vi "Test Collection.vi"(8 "error in (no error)":errorcluster) -> (0 "error out":errorcluster)   [LabVIEW 2020]
uses:
  cc2f4b2e-6b9b-4032-8eb1-861370e43379.vi
  70896fcf-518f-4248-9f1c-0e40431e55ec.vi
  c8c48edb-c7f5-472d-977d-3a0b36aefcc9.vi
  3ab85443-7e8d-4878-a956-06c51692e772.vi
  e6d767b0-dcee-4f8d-a596-45b7e0fa1c6e.vi
  ad483bc9-2563-4378-ab89-dc41a6632da3.vi
  1ba9e6c7-e427-431f-8c56-b87e95f623b9.vi
  <vilib>/addons/_JKI Toolkits/Caraya/classes/Assert/Assert.lvclass
  <vilib>/addons/_JKI Toolkits/Caraya/classes/Test/Test.lvclass
  <vilib>/addons/_JKI Toolkits/Caraya/classes/Assert/Assert Equal Value and Type_Variant.vi
  b04bc5c7-8eec-4582-9321-dcd999a304b5.vi
  4da1d838-1536-4b81-8938-06410ac1efc2.vi
  09fb3b3b-0f42-404c-85cb-5df9e4b15e48.vi
  <vilib>/addons/_JKI Toolkits/Caraya/classes/Assert/Assert Equal Type_Variant.vi
  135354c9-91d1-468c-a7ac-d8cf1757bf8f.vi
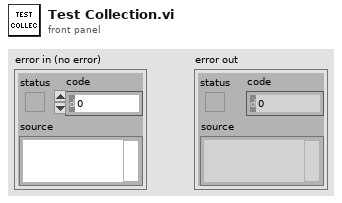
[diagram p1: front panel]
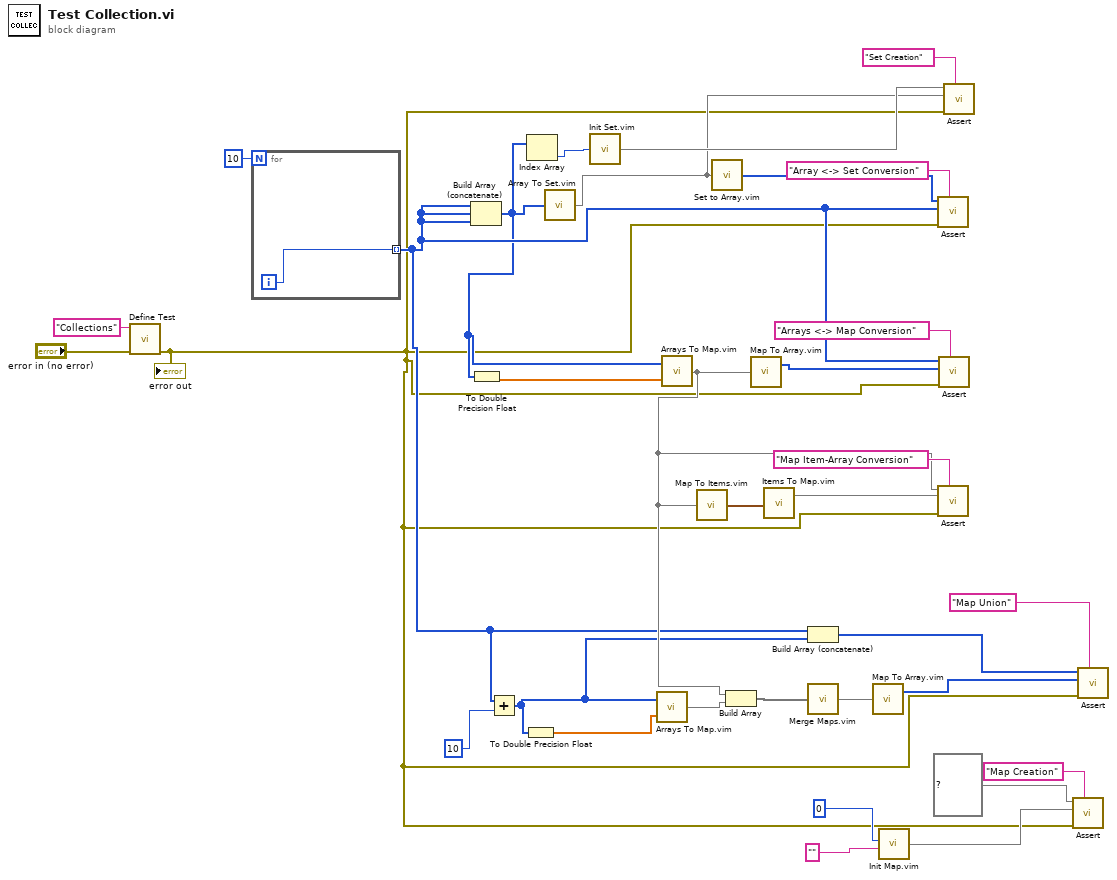
[diagram p0: block diagram]
diagram:
  n1 = call <vilib>:"Define Test.vi"("error in (no error)"="error in (no error)", "Label (VI Title)"="Collections") -> ("error out"=w3:errorcluster)  [unwired: 9 in]
  "error out" <- w3
  n2 = for {
    N: 10 -> [_]
    tunnel: [w34] -> w13 mode=indexing
    i -> [w34]
  }
  n3 = Build Array (concatenate)(w13, w13, w13) -> (w7:i32[])
  n4 = To Double Precision Float(number=w7) -> (double precision float=w30:dbl[])
  n5 = Add(x=w13, y=10) -> (x+y=w17:i32[])
  n6 = To Double Precision Float(number=w17) -> (double precision float=w20:dbl[])
  n7 = Index Array(array=w7) -> (element=w6:i32)  [unwired: 1 in]
  n8 = call "Array To Set.vim"("Array"=w7) -> ("set"=w4:set{i32})
  n9 = call "Init Set.vim"("Type"=w6) -> ("Empty Set"=w5:set{i32})
  n10 = call "Arrays To Map.vim"("Values"=w20, "Keys"=w17) -> ("map"=w23:map{i32, dbl})
  n11 = call "Arrays To Map.vim"("Values"=w30, "Keys"=w7) -> ("map"=w22:map{i32, dbl})
  n12 = call "Map To Items.vim"("Map"=w22) -> ("Items"=w26:cluster{"key":i32, "value":dbl}[])
  n13 = call "Set to Array.vim"("Set"=w4) -> ("Array"=w31:i32[])
  n14 = Build Array(w22, w23) -> (w19:map{i32, dbl}[])
  n15 = call "Map To Array.vim"("Map"=w22) -> ("Keys"=w28:i32[])  [unwired: 1 out]
  n16 = call "Items To Map.vim"("Items"=w26) -> ("Map"=w25:map{i32, dbl})  [unwired: 1 out]
  n17 = Build Array (concatenate)(w13, w17) -> (w16:i32[])
  n18 = call "Merge Maps.vim"("Map In"=w19) -> ("Merged Maps"=w18:map{i32, dbl})
  n19 = call "Map To Array.vim"("Map"=w18) -> ("Keys"=w15:i32[])  [unwired: 1 out]
  n20 = call "Init Map.vim"("Key Type"=0, "Value type"="") -> ("map out"=w9:map{variant, variant})  [unwired: 6 in]
  n21 = call-poly <vilib>:"Assert.vi"("Label"="Array <-> Set Conversion", "error in (no error)"=w3, "Y"=w13, "X"=w31) -> ()  [unwired: 7 in, 1 out]
  n22 = call-poly <vilib>:"Assert.vi"("Label"="Map Item-Array Conversion", "error in (no error)"=w3, "Y"=w25, "X"=w22) -> ()  [unwired: 7 in, 1 out]
  n23 = call-poly <vilib>:"Assert.vi"("Label"="Arrays <-> Map Conversion", "error in (no error)"=w3, "Y"=w28, "X"=w13) -> ()  [unwired: 7 in, 1 out]
  n24 = call-poly <vilib>:"Assert.vi"("Label"="Set Creation", "error in (no error)"=w3, "Y"=w4, "X"=w5) -> ()  [unwired: 7 in, 1 out]
  n25 = call-poly <vilib>:"Assert.vi"("Label"="Map Creation", "error in (no error)"=w3, "Y"=w9, "X"=map{i32, string} {} ("Empty Map out")) -> ()  [unwired: 7 in, 1 out]
  n26 = call-poly <vilib>:"Assert.vi"("Label"="Map Union", "error in (no error)"=w3, "Y"=w15, "X"=w16) -> ()  [unwired: 7 in, 1 out]
